vi "Queue Actor.vi"(10 "Spawn":refnum<class "Spawn.lvclass">, 11 "TEMPLATE Actor in":refnum<class "TEMPLATE Actor.lvclass">) -> (0 "Error out":errorcluster, 3 "TEMPLATE Actor out":refnum<class "TEMPLATE Actor.lvclass">)   [LabVIEW 2025, in "_Template.lvlib" / "Templates.lvlib" / "TEMPLATE Actor.lvlib" / "TEMPLATE Actor.lvclass"]
uses:
  TEMPLATE Actor.lvclass
  TEMPLATE Actor.lvclass/TEMPLATE Actor.ctl
  jettl/jettl/jettl.lvlib
  jettl/jettl/Transport/Queue/Queue.lvlib
  Control Refs.ctl
  jettl/jettl/Spawn/Spawn/Spawn.lvclass
types:
  T1 = typedef "_Template.lvlib/Templates.lvlib/TEMPLATE Actor.lvlib/TEMPLATE Actor.lvclass/Control Refs.ctl" = cluster{}
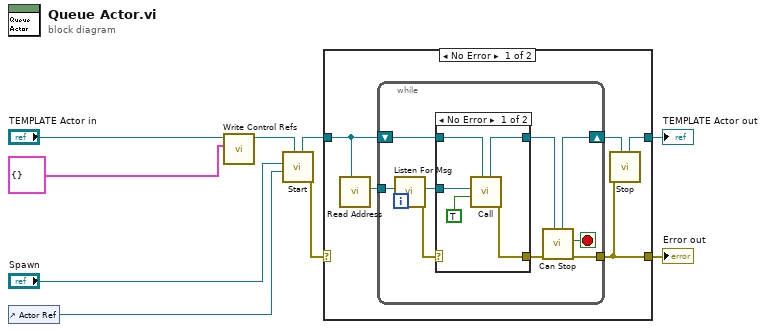
[diagram p0: block diagram]
diagram:
  n1 = control-ref of="Actor Ref"() -> (w5:refnum<vi>)
  n2 = call "Write Control Refs.vi"("Control Refs"=T1 {} ("Process Refs"), "TEMPLATE Actor in"="TEMPLATE Actor in") -> ("TEMPLATE Actor out"=w2:refnum<class "TEMPLATE Actor.lvclass">)  [unwired: 9 in]
  n3 = call "Start.vi"("Actor in"=w2, "Actor Ref"=w5, "Spawn"="Spawn") -> ("Error out"=w7:errorcluster, "Actor out"=w6:refnum<class "TEMPLATE Actor.lvclass">)  [unwired: 7 in]
  n4 = case shown="No Error" w7 {
    selector: w7 -> [_ w31]
    tunnel: [w12 w32] -> w9
    tunnel: w6 -> [w11 w32]
    tunnel: [w14 w31] -> w8
    frame No Error {
      n5 = call "Read Address.vi"("Actor"=w11) -> ("Address"=w10:refnum<data-value>)  [unwired: 10 in]
      n6 = while {
        shift-right: [w21] -> w13
        shift-left: w11 -> [w19]
        tunnel: [w22] -> w14
        tunnel: w10 -> [w17]
        stop <- w20 stop-if-true
        n7 = call "Listen For Msg.vi"("Address"=w17) -> ("Error out"=w15:errorcluster, "Msg"=w16:refnum<class "Msg.lvclass">)  [unwired: 9 in]
        n8 = case shown="No Error" w15 {
          selector: w15 -> [_ w29]
          tunnel: [w28 w29] -> w23
          tunnel: w19 -> [w27 w30]
          tunnel: [w26 w30] -> w18
          tunnel: w16 -> [w25 _]
          frame No Error {
            n9 = call "Call.vi"("Actor in"=w27, "Listened To Msg"=TRUE, "Msg"=w25) -> ("Error out"=w28:errorcluster, "Actor out"=w26:refnum<class "TEMPLATE Actor.lvclass">)  [unwired: 6 in, 1 out]
          }
          frame Error {
          }
        }
        n10 = call "Can Stop.vi"("Actor in"=w18, "Error in"=w23) -> ("Error out"=w22:errorcluster, "Stop"=w20:bool, "Actor out"=w21:refnum<class "TEMPLATE Actor.lvclass">)  [unwired: 7 in]
      }
      n11 = call "Stop.vi"("Actor in"=w13, "Error in"=w14) -> ("Actor out"=w12:refnum<class "TEMPLATE Actor.lvclass">)  [unwired: 9 in]
    }
    frame Error {
    }
  }
  "TEMPLATE Actor out" <- w9
  "Error out" <- w8
